vi "remove empty elements.vi"(10 "array in":string[](array[string])) -> (2 "array without blanks out":string[](array[string]))   [LabVIEW 2020, in "stream_custom_cluster.lvclass"]
uses:
  stream_custom_cluster.lvclass
  stream_custom_cluster.lvclass/stream_custom_cluster.ctl
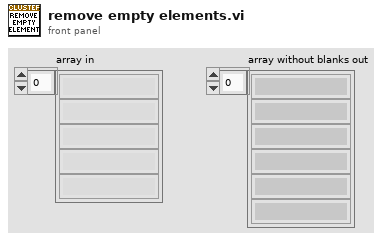
[diagram p1: front panel]
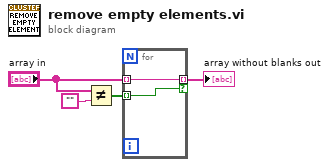
[diagram p0: block diagram]
diagram:
  n1 = Not Equal?(x="array in", y="") -> (x != y?=w2:bool[])
  n2 = for {
    tunnel: [w6] -> w1 mode=indexing if=w5
    tunnel: "array in" -> [w6] mode=indexing
    tunnel: w2 -> [w5] mode=indexing
  }
  "array without blanks out" <- w1
